vi "Read Heap Save Format.vi"(8 "error in (no error)":errorcluster) -> (0 "error out":errorcluster, 3 "Heap Save Format":T1=1 items=["Off", "XML", "Binary", "Verbose Tagged Text", "Binary2"])   [LabVIEW 2026, in "VILab.lvlib"]
uses:
  VILab.lvlib
  CTLs/Heap Save Format.ctl
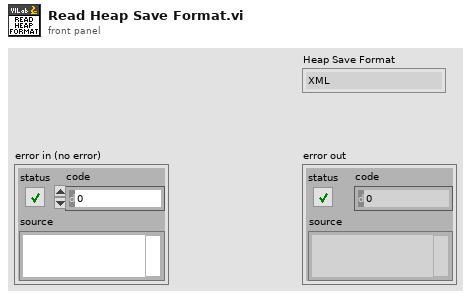
[diagram p1: front panel]
types:
  T1 = typedef "VILab.lvlib/Heap Save Format.ctl" = u16
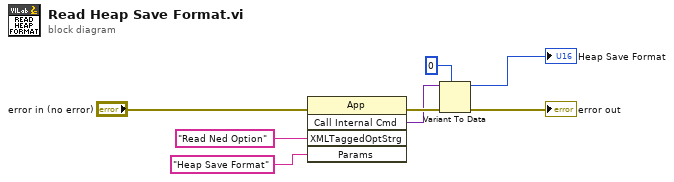
[diagram p0: block diagram]
diagram:
  n1 = invoke class="App" method="Call Internal Cmd"(error in="error in (no error)", "XMLTaggedOptStrg"="Read Ned Option" ("Command Name"), "Params"="Heap Save Format") -> (error out=w8:errorcluster, "CallInternalCmd"=w5:variant)  [unwired: 2 in, 3 out]
  n2 = Variant To Data(error in=w8, type=0, Variant=w5) -> (data=→"Heap Save Format":i32, error out=→"error out":errorcluster)
